vi "SENS_CORR_STAT_ON_OFF.vi"(0 "VISA IN":refnum<visa-resource-name>, 1 "Correction Applied ON/OFF":bool, 5 "error in":errorcluster, 7 "Channel":i32) -> (14 "VISA Out":refnum<visa-resource-name>, 19 "error out":errorcluster)   [LabVIEW 2018, in "PNA-X.lvlib"]
doc: "SENSe<cnum>:CORRection[:STATe] <ON | OFF> \n1639\n\n(Read-Write) Turns error correction ON and OFF for the specified channel. \nNote: Before using this command you must select a measurement using CALC:PAR:SEL. You can \nselect one measurement for each channel. \nParameters \n<cnum> Any existing channel number. If unspecified, value is set to 1 \n<ON | OFF> ON (or 1) - correction is applied to the channel. \nOFF (or 0) - correction is NOT applied to the channel. \nExamples SENS:CORR ON \nsense2:correction:state off \nQuery Syntax SENSe<cnum>:CORRection[:STATe]? \nTo query the error correction state for a measurement, use CALC:CORR:STATe? \nReturn Type Boolean (1 = ON, 0 = OFF) \nDefault OFF \nSENSe:CORRection:TSTandards[:STATe] <boolean> \n(Read-Write) Specifies the acquisition of calibration data using ONE or TWO sets of standards. \nParameters \n<boolean> ON (1) - TWO identical sets of standards will be used to simultaneously \ncalibrate two ports (for both Forward and Reverse parameters). \nOFF (0)- ONE set of standards will be used to perform a full 2-port calibration, \none port at a time. \nWhen specifying ON (use two sets), the SENS:CORR:COLL:ACQuire \ncommand uses the same standard index for each calibration class. To specify \nthe calibration standard gender for each port, you must first ensure that the \norder of calibration class accurately reflects the configuration of your DUT. \nFor example, for a DUT with a male connector on port 1 and a female \nconnector on port 2, order the devices within the S11 classes (A, B, and C) \nsuch that the MALE standards are first in the list. Then order the S22 classes \nspecifying the FEMALE standards as the first in the list. \nExamples SENS:CORR:TST 1 \nsense:correction:tstandard:state 0 \nSee an example using this command \n1640\n\nQuery Syntax SENSe:CORRection:TSTandards[:STATe]? \nReturn Type Boolean \nDefault ON \nSENSe:CORRection:TYPE:CATalog? <char> \n(Read-Write) Lists the Cal Types in the PNA by either GUID or registered name. Learn more about \napplying Cal Type using SCPI. \nNote: Before using this command you must select a measurement using CALC:PAR:SEL. You can \nselect one measurement for each channel. \nParameters \n<char> Specifies the type of list. Choose from: \nGUID - the registered GUID of the Cal Type \nNAME - the registered name of the Cal Type \nExamples SENS:CORR:TYPE:CAT? GUID \nQuery Syntax SENSe<cnum>:CORRection:TYPE:CATalog? <char> \nReturn Type Comma-separated string \nDefault Not Applicable \nLast modified: \nApril 14, \n2007 \nAddd ECal isolation commands \nOct 30, \n2006 \nModified SavUser command \n1641\n\nSense:Correction:Collect:Guided Commands \nPerforms and applies a SmartCal (Guided) calibration and other error correction features. \nClick on a blue keyword to view the command details. \nSee Also \nExamples using these commands. \n1642\n\nNew Calibrating the PNA Using SCPI \nLearn about Measurement Calibration \nSynchronizing the PNA and Controller \nSENSe:CORRection:COLLect:GUIDed:ACQuire <std> \n(Write-only) Initiates the measurement of the specified calibration standard. Executing this command \nwith an unnecessary standard has no affect. \nThe measured data is stored and used for subsequent calculations of error correction coefficients. All \nstandards must be measured before a calibration can be completed. Any measurement can be repeated \nuntil the SENS:CORR:COLL:GUID:SAVE command is executed. \nQuery the user prompt description using SENS:CORR:COLL:GUID:DESC? \nQuery the required calibration steps using SENS:CORR:COLL:GUID:STEP? \nParameters \n<cnum> Any existing channel number. If unspecified, value is set to 1 \n<std> Choose from:STAN1, STAN2, STAN3, through STAN40 \nExamples SENS:CORR:COLL:GUID:ACQ STAN1 \nsense:correction:collect:guided:acquire stan1 \nQuery Syntax Not Applicable \nDefault Not Applicable"
uses:
  PNA-X.lvlib
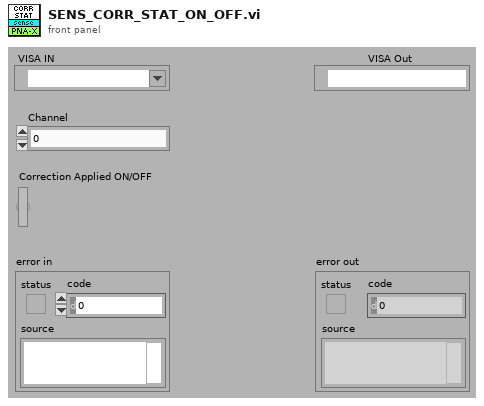
[diagram p1: front panel]
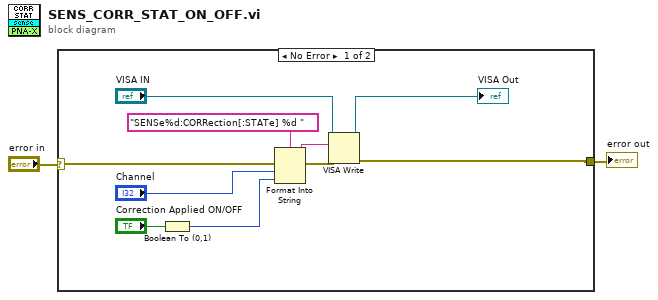
[diagram p0: block diagram]
diagram:
  n1 = case shown="No Error" "error in" {
    selector: "error in" -> [w12 w13]
    tunnel: [w7 w13] -> w1
    frame No Error {
      n2 = Boolean To (0,1)(Boolean="Correction Applied ON/OFF") -> (0, 1=w3:i16)
      n3 = Format Into String(format string="SENSe%d:CORRection[:STATe] %d " ("Cmdline"), error in=w12, "Channel", w3) -> (resulting string=w10:string, error out=w11:errorcluster)  [unwired: 1 in]
      n4 = VISA Write(VISA resource name="VISA IN", write buffer=w10, error in (no error)=w11) -> (VISA resource name out=→"VISA Out":refnum<visa-resource-name>, error out=w7:errorcluster)  [unwired: 1 out]
    }
    frame Error {
    }
  }
  "error out" <- w1
